vi "Tosca-Start Synapse Recording.vi"(0 "Path":path, 11 "error in (no error)":errorcluster) -> (4 "Path out":path, 15 "error out":errorcluster)   [LabVIEW 2020]
uses:
  Typedefs/Tosca-Synapse Settings.ctl
  Tosca-Globals.vi
  <vilib>/regexp/Match Regular Expression.xnode
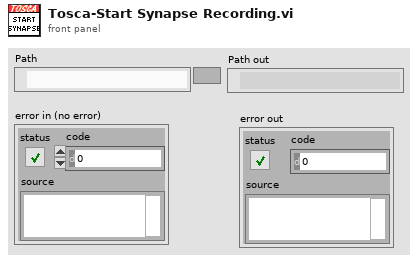
[diagram p1: front panel]
types:
  T1 = enum16{"big-endian, network order", "native, host order", "little-endian"}
  T2 = typedef "Tosca-Synapse Settings.ctl" = cluster{"IP Address":string, "Port":i32, "Record timeout (ms)":i32}
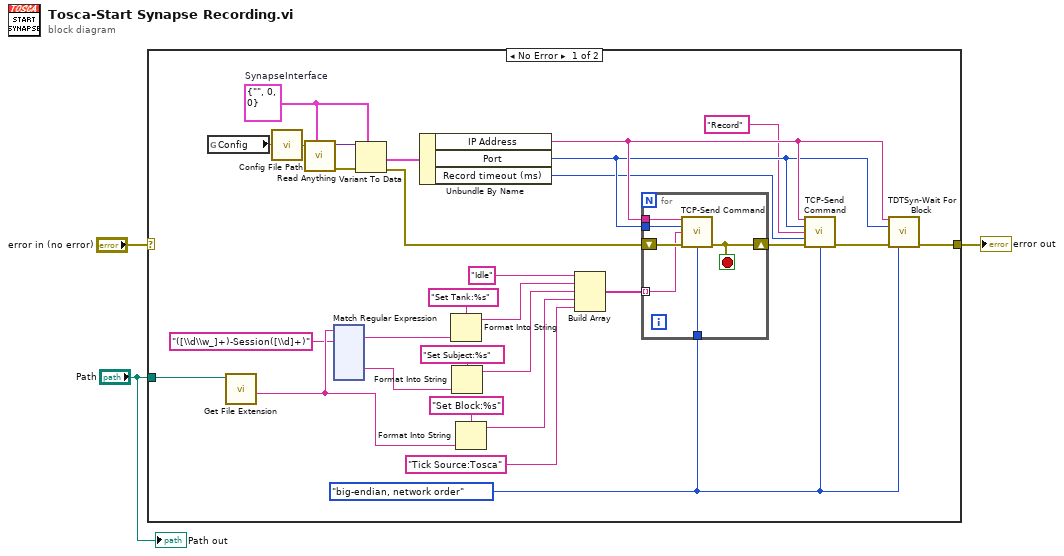
[diagram p0: block diagram]
diagram:
  n1 = case shown="No Error" "error in (no error)" {
    selector: "error in (no error)" -> [_ w156]
    tunnel: [w14 w156] -> w2
    tunnel: "Path" -> [w25 _]
    frame No Error {
      w4 = T1."big-endian, network order" ("byte order")
      w11 = T2 {"IP Address"="", "Port"=0, "Record timeout (ms)"=0}  # SynapseInterface
      n2 = global read "Tosca-Globals.vi" "Config"() -> (w12:string)
      n3 = call <vilib>:"Get File Extension.vi"("file"=w25) -> ("filename without extension"=w20:string)  [unwired: 6 in, 4 out]
      n4 = call "Config File Path.vi"("AppName"=w12) -> ("Default config file name"=w32:path)
      n5 = call "Read Anything.vi"("Type of Anything"=w11, "Path (dialog)"=w32) -> ("Error Out"=w30:errorcluster, "Anything"=w31:variant)  [unwired: 7 in, 1 out]
      n6 = xnode "Match Regular Expression"("input string"=w20, "regular expression"="([\\d\\w_]+)-Session([\\d]+)") -> ("whole match"=w18:string, "submatch 1"=w16:string)  [unwired: 4 in, 5 out]
      n7 = Variant To Data(error in=w30, type=w11, Variant=w31) -> (data=w29:T2, error out=w28:errorcluster)
      n8 = Unbundle By Name(w29) -> ("IP Address"=w8:string, "Port"=w7:i32, "Record timeout (ms)"=w6:i32)
      n9 = Format Into String(format string="Set Tank:%s", w18) -> (resulting string=w23:string)  [unwired: 2 in, 1 out]
      n10 = Format Into String(format string="Set Subject:%s", w16) -> (resulting string=w15:string)  [unwired: 2 in, 1 out]
      n11 = Format Into String(format string="Set Block:%s", w20) -> (resulting string=w22:string)  [unwired: 2 in, 1 out]
      n12 = Build Array("Idle" ("Command"), w23, w15, w22, "Tick Source:Tosca" ("Command")) -> (w21:string[])
      n13 = for {
        tunnel: w8 -> [w38]
        tunnel: w7 -> [w37]
        shift-right: [w34] -> w10
        shift-left: w28 -> [w36]
        tunnel: w21 -> [w35] mode=indexing
        tunnel: w4 -> [w33]
        stop <- w34 stop-if-true
        n14 = call "TCP-Send Command.vi"("PXI Address"=w38, "Port"=w37, "Command"=w35, "error in (no error)"=w36, "byte order"=w33) -> ("error out"=w34:errorcluster)  [unwired: 10 in]
      }
      n15 = call "TCP-Send Command.vi"("PXI Address"=w8, "Port"=w7, "Command"="Record", "timeout (ms)"=w6, "error in (no error)"=w10, "byte order"=w4) -> ("error out"=w9:errorcluster)  [unwired: 9 in]
      n16 = call "TDTSyn-Wait For Block.vi"("IP Address"=w8, "Port"=w7, "error in (no error)"=w9, "byte order"=w4) -> ("error out"=w14:errorcluster)  [unwired: 11 in]
    }
    frame Error {
    }
  }
  "error out" <- w2
  "Path out" <- "Path"
